vi "DBM_WorkInProg.vi"(8 "error in (no error)":errorcluster, 11 "DBManager in":refnum<class "DBManager.lvclass">) -> (0 "error out":errorcluster, 2 "Work in progress?":bool, 3 "DBManager out":refnum<class "DBManager.lvclass">)   [LabVIEW 2015, in "DBManager.lvclass"]
uses:
  DBManager.lvclass
  DBManager.lvclass/DBManager.ctl
  <vilib>/drjdpowell/SQLite Library/SQL Statement/SQL Statement.lvclass/SQL Statement.ctl
  <vilib>/drjdpowell/SQLite Library/SQL Statement/Column I64.vi
  <vilib>/drjdpowell/SQLite Library/SQL Statement/Error Message.vi
  <vilib>/drjdpowell/SQLite Library/SQL Statement/SQL Statement.lvclass
  <vilib>/drjdpowell/SQLite Library/SQL Connection/Connection.lvclass
panel:
  # "Connector Pane"
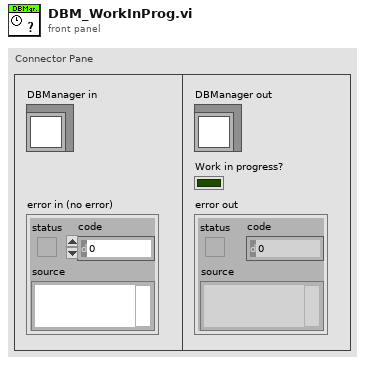
[diagram p1: front panel]
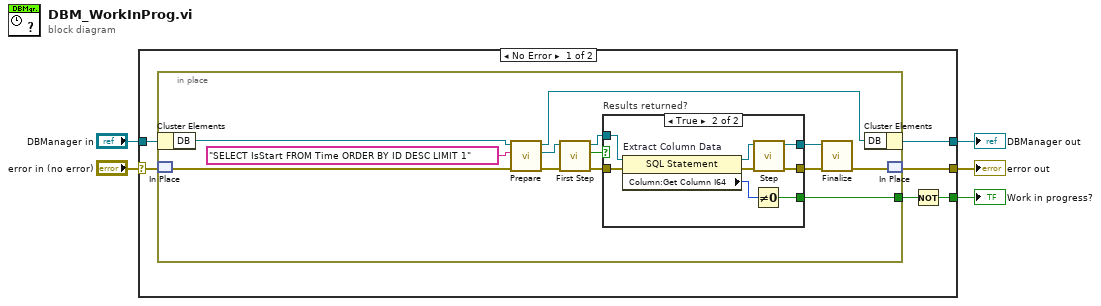
[diagram p0: block diagram]
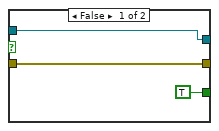
[diagram p2: hidden frame]
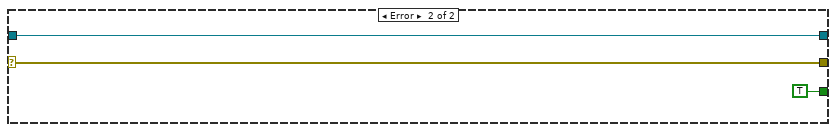
[diagram p3: hidden frame]
diagram:
  n1 = case shown="No Error" "error in (no error)" {
    selector: "error in (no error)" -> [w10 w38]
    tunnel: [w8 w38] -> w3
    tunnel: [w9 w37] -> w2
    tunnel: "DBManager in" -> [w11 w37]
    tunnel: [w6 TRUE] -> w1
    frame No Error {
      n2 = in-place {
        in-place-border: [w12] -> w7
        n3 = in-place-cluster #1(w11) -> ("DB"=w13:refnum<class "Connection.lvclass">)
        n4 = in-place-match #2(w10) -> (w16:errorcluster)
        n5 = call <vilib>:"Prepare.vi"("error in (no error)"=w16, "SQL"="SELECT IsStart FROM Time ORDER BY ID DESC LIMIT 1" ("SELECT  statement"), "SQLite Connection in"=w13) -> ("error out"=w20:errorcluster, "SQL Statement out"=w21:refnum<class "SQL Statement.lvclass">, "SQLite Connection out"=w14:refnum<class "Connection.lvclass">)  [unwired: 4 in, 2 out]
        n6 = call <vilib>:"First Step.vi"("error in (no error)"=w20, "SQL Statement in"=w21) -> ("error out"=w23:errorcluster, "Row returned"=w24:bool, "SQL Statement out"=w22:refnum<class "SQL Statement.lvclass">)  [unwired: 7 in]
        n7 = case "Results returned?" shown="True" w24 {
          tunnel: [w27 w35] -> w18
          tunnel: [w26 w34] -> w17
          tunnel: w22 -> [w27 w33]
          tunnel: w23 -> [w26 w32]
          tunnel: [TRUE w28] -> w12
          frame False {
          }
          frame True {
            n8 = property on="Extract Column Data" class="SQL Statement"(reference=w33, error in=w32) -> (reference out=w31:refnum<class "SQL Statement.lvclass">, error out=w30:errorcluster, "Column:Get Column I64"=w29:i64)
            n9 = Not Equal To 0?(x=w29) -> (x != 0?=w28:bool)
            n10 = call <vilib>:"Step.vi"("error in (no error)"=w30, "SQL Statement in"=w31) -> ("error out"=w34:errorcluster, "SQL Statement out"=w35:refnum<class "SQL Statement.lvclass">)  [unwired: 7 in, 1 out]
          }
        }
        n11 = call <vilib>:"Finalize.vi"("error in (no error)"=w17, "SQL Statement in"=w18) -> ("error out"=w15:errorcluster)  [unwired: 9 in]
        n12 = in-place-cluster #1("DB"=w14) -> (w9:refnum<class "DBManager.lvclass">)
        n13 = in-place-match #2(w15) -> (w8:errorcluster)
      }
      n14 = Not(x=w7) -> (.not. x?=w6:bool)
    }
    frame Error {
    }
  }
  "error out" <- w3
  "DBManager out" <- w2
  "Work in progress?" <- w1
